vi "Set Continuous Sweep Attributes.vi"(5 "Profile":u16(ring)=1 items=["Linear", "Logarithmic"], 7 "Duration":dbl, 9 "stop":dbl=10000.0 format="%.2f", 10 "start":dbl=10.0 format="%.2f", 11 "Display State Attributes in":variant) -> (2 "name":string="ContinuousSweepInfo", 3 "Display State Attributes out":variant)   [LabVIEW 2017, in "Test Signal Configuration.xctl"]
uses:
  <vilib>/addons/_XControls/Function Generator Configuration/Test Signal Configuration.xctl
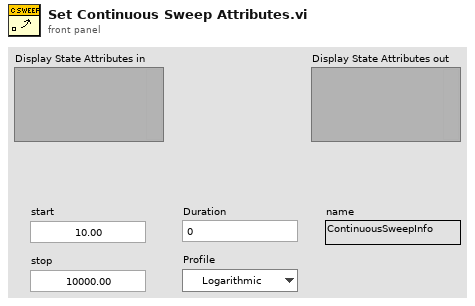
[diagram p1: front panel]
types:
  T1 = typedef "Test Signal Configuration.xctl/signal type.ctl" = enum32{"None", "Tone", "Multitone", "Discrete Sweep", "Continuous Sweep", "Noise"}
  T2 = cluster{"Signal":cluster{"Sample Rate":cluster{"name":string, "default":dbl}, "Signal Type":cluster{"name":string, "signal type":T1}, "Amplitude":cluster{"name":string, "default":dbl}, "Offset":cluster{"name":string, "default":dbl}}, "Function":cluster{"Info":cluster{"name":string, "default":variant}, "Type":cluster{"name":string, "default":u16}, "Frequency":cluster{"name":string, "default":dbl}, "Phase":cluster{"name":string, "default":dbl}}, "Continuous Sweep":cluster{"Info":cluster{"name":string, "default":variant}, "Start":cluster{"name":string, "default":dbl}, "Stop":cluster{"name":string, "default":dbl}, "Duration":cluster{"name":string, "default":dbl}, "Profile":cluster{"name":string, "default":enum16{"Linear", "Logarithmic"}}}, "Discrete Sweep":cluster{"Info":cluster{"name":string, "default":variant}, "Start":cluster{"name":string, "default":dbl}, "Stop":cluster{"name":string, "default":dbl}, "Cycles":cluster{"name":string, "default":dbl}, "Time":cluster{"name":string, "default":dbl}, "Spacing":cluster{"name":string, "default":enum16{"Linear", "Logarithmic"}}, "Steps":cluster{"name":string, "default":i32}}, "Multitone":cluster{"Info":cluster{"name":string, "multitone info":cluster{"frequency":dbl, "amplitude":dbl, "phase":dbl}[]}}, "Noise":cluster{"Info":cluster{"name":string, "default":variant}, "Type":cluster{"name":string, "default":u16}, "Amplitude PDF":cluster{"name":string, "default":enum16{"Gaussian", "Rectangular", "Triangular"}}, "Level":cluster{"name":string, "default":dbl}, "Seed":cluster{"name":string, "default":i32}}, "Configuration":cluster{"Min Frequency":cluster{"name":string, "default":dbl}, "Max Frequency":cluster{"name":string, "default":dbl}, "Max Amplitude":cluster{"name":string, "default":dbl}}}
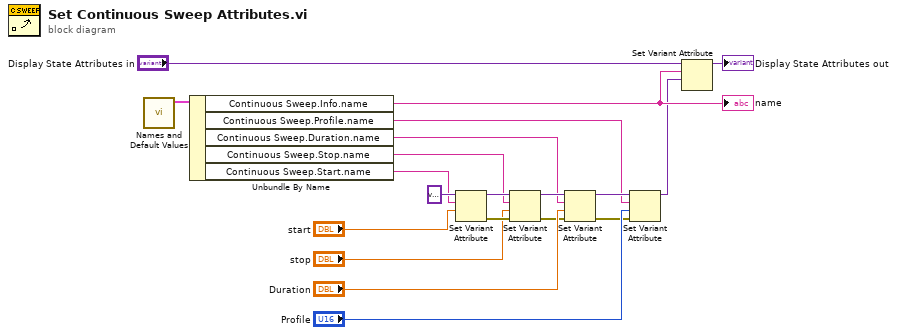
[diagram p0: block diagram]
diagram:
  n1 = call <vilib>:"Names and Default Values.vi"() -> ("Names and Default Values"=w11:T2)  [unwired: 11 in]
  n2 = Unbundle By Name(w11) -> ("Continuous Sweep.Info.name"=w2:string, "Continuous Sweep.Profile.name"=w10:string, "Continuous Sweep.Duration.name"=w9:string, "Continuous Sweep.Stop.name"=w8:string, "Continuous Sweep.Start.name"=w7:string)
  "name" <- w2
  n3 = Set Variant Attribute(Variant=variant, name=w7, value="start") -> (Variant out=w13:variant, error out=w12:errorcluster)  [unwired: 1 in, 1 out]
  n4 = Set Variant Attribute(Variant=w13, name=w8, value="stop", error in=w12) -> (Variant out=w17:variant, error out=w16:errorcluster)  [unwired: 1 out]
  n5 = Set Variant Attribute(Variant=w17, name=w9, value="Duration", error in=w16) -> (Variant out=w15:variant, error out=w14:errorcluster)  [unwired: 1 out]
  n6 = Set Variant Attribute(Variant=w15, name=w10, value="Profile", error in=w14) -> (Variant out=w1:variant)  [unwired: 2 out]
  n7 = Set Variant Attribute(Variant="Display State Attributes in", name=w2, value=w1) -> (Variant out=→"Display State Attributes out":variant)  [unwired: 1 in, 2 out]
